vi "Double IsEqual.vi"(9 "Epsilon":dbl, 10 "Double2":dbl, 11 "Double1":dbl) -> (3 "IsEqual":bool)   [LabVIEW 2012]
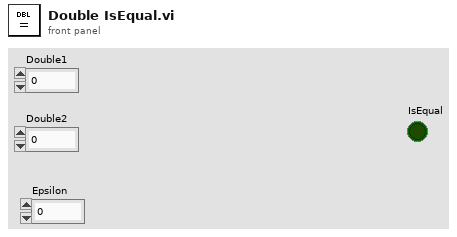
[diagram p1: front panel]
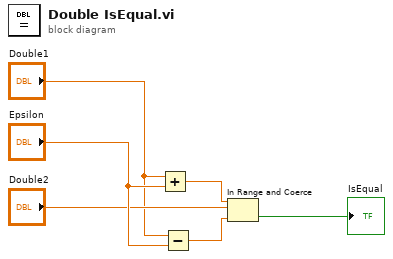
[diagram p0: block diagram]
diagram:
  n1 = Add(x="Double1", y="Epsilon") -> (x+y=w6:dbl)
  n2 = Subtract(x="Double1", y="Epsilon") -> (x-y=w3:dbl)
  n3 = In Range and Coerce(upper limit=w6, x="Double2", lower limit=w3) -> (In Range?=→"IsEqual":bool)  [unwired: 1 out]
